vi "test_Create Periodic & Trigger Message.vi"(8 "error in (no error)":errorcluster, 11 "TestCase in":refnum<class "Instrument Addon Scripting API Messages Unit Tests.lvclass">) -> (0 "error out":errorcluster, 3 "TestCase out":refnum<class "Instrument Addon Scripting API Messages Unit Tests.lvclass">)   [LabVIEW 2019, in "Instrument Addon Scripting API Messages Unit Tests.lvclass"]
uses:
  Instrument Addon Scripting API Messages Unit Tests.lvclass
  <vilib>/addons/_JKI Toolkits/VI Tester/TestCase.llb/TestCase.lvclass
  APIs/Scripting API/Instrument Addon Scripting API.lvlib
  NationalInstruments.VeriStand.SystemDefinitionAPI
  <vilib>/NI VeriStand/Custom Device Tools/Custom Device Utility Library/Custom Device Utility Library.lvlib
  Addon/Addon Shared/SubVIs/Constants.vi
  Addon/Addon Shared/Instrument Addon Shared.lvlib
  APIs/Scripting API/TypeDefs/Protection Types.ctl
  APIs/Scripting API/TypeDefs/Message Settings.ctl
  Addon/Addon Shared/Types/FG Control.ctl
  Addon/Addon Shared/Types/Message Generation Type.ctl
  APIs/Scripting API/Messages/Create Message - Periodic & Trigger.vi
  <vilib>/NI VeriStand/Custom Device Tools/Custom Device Utility Library/NI VeriStand - Search for Item by GUID.vi
  C:/Program Files (x86)/National Instruments/LabVIEW 2019/vi.lib/addons/_JKI Toolkits/VI Tester/TestCase.llb/TestCase.lvclass
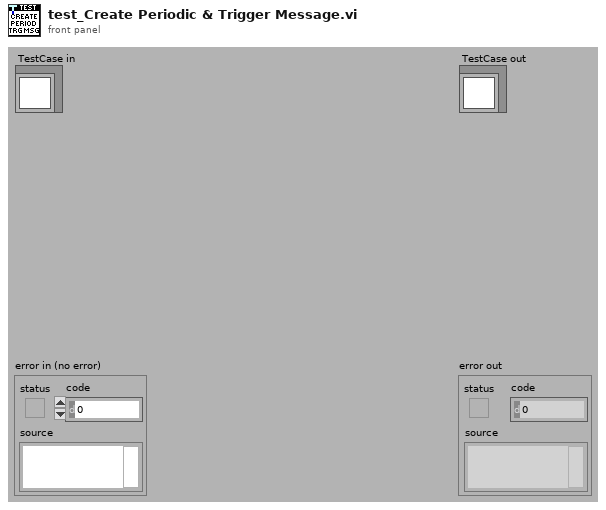
[diagram p1: front panel]
types:
  T1 = typedef "Instrument Addon Shared.lvlib/FG Control.ctl" = enum16{"Get", "Set"}
  T2 = typedef "Instrument Addon Shared.lvlib/Message Generation Type.ctl" = enum16{"Trigger Only", "Periodic & Trigger", "Value Change & Trigger"}
  T3 = typedef "Instrument Addon Scripting API.lvlib/Message Settings.ctl" = cluster{"Protection":T4, "Enable Periodic Default":bool, "Trigger Channel refnum":u64}
  T4 = typedef "Instrument Addon Scripting API.lvlib/Protection Types.ctl" = enum16{"None", "CRC-32", "Checksum U16", "Checksum U32", "Checksum U8"}
  T5 = typedef "Custom Device API.lvlib/Custom Device Item Ref.ctl" = u64
  T6 = typedef "Instrument Addon Shared.lvlib/Trigger Parameters.ctl" = cluster{"Use Channel":bool, "Channel Path":string}
  T7 = typedef "Instrument Addon Shared.lvlib/Message Parameters.ctl" = cluster{"Generation Type":T2, "Period":dbl, "Include Protection":bool, "Type":string}
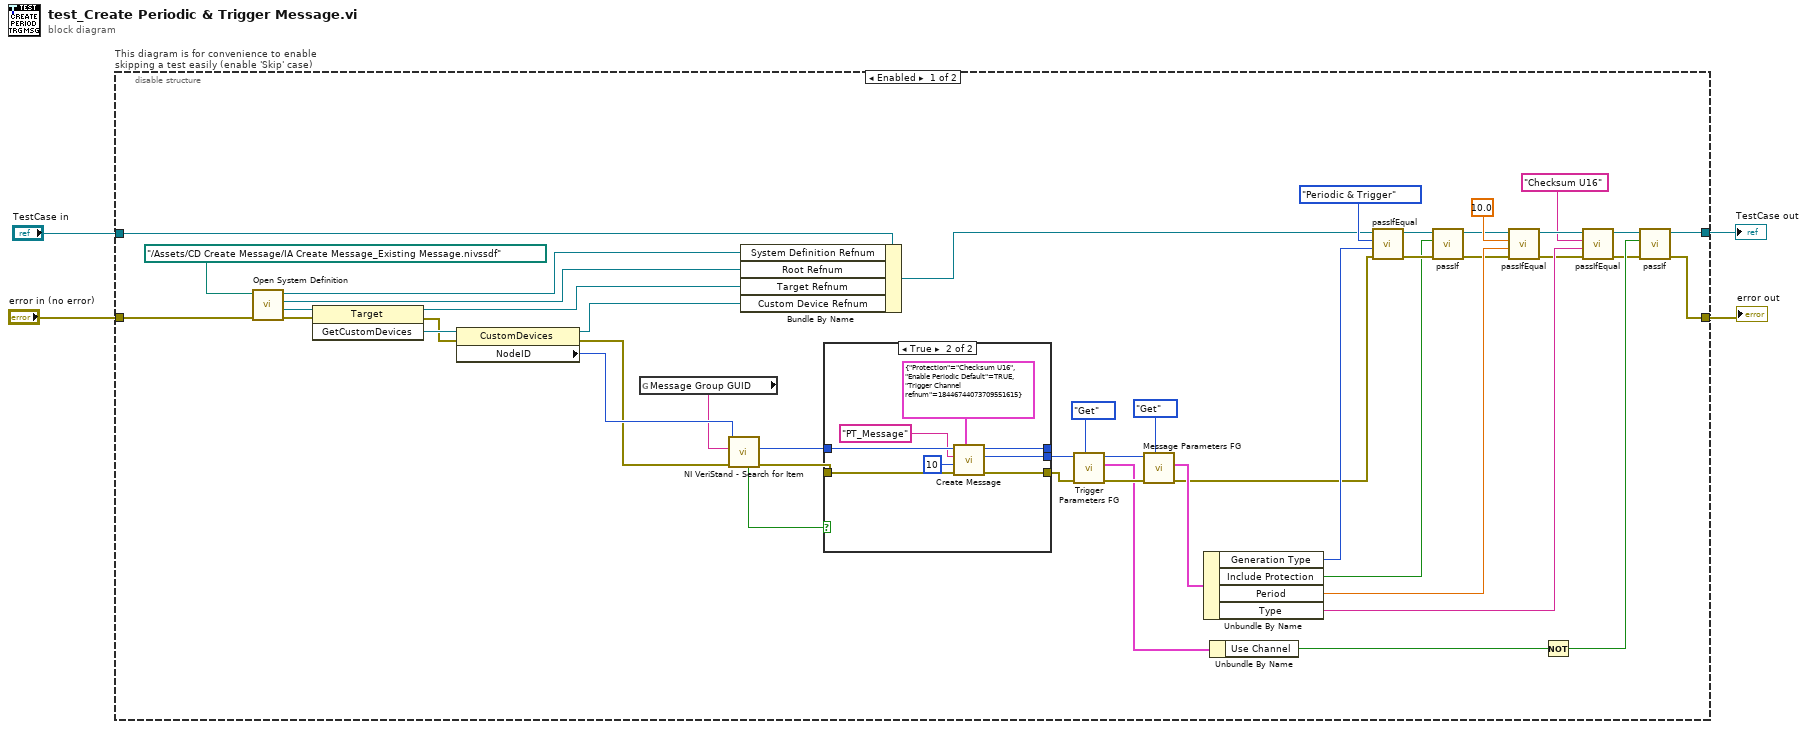
[diagram p0: block diagram]
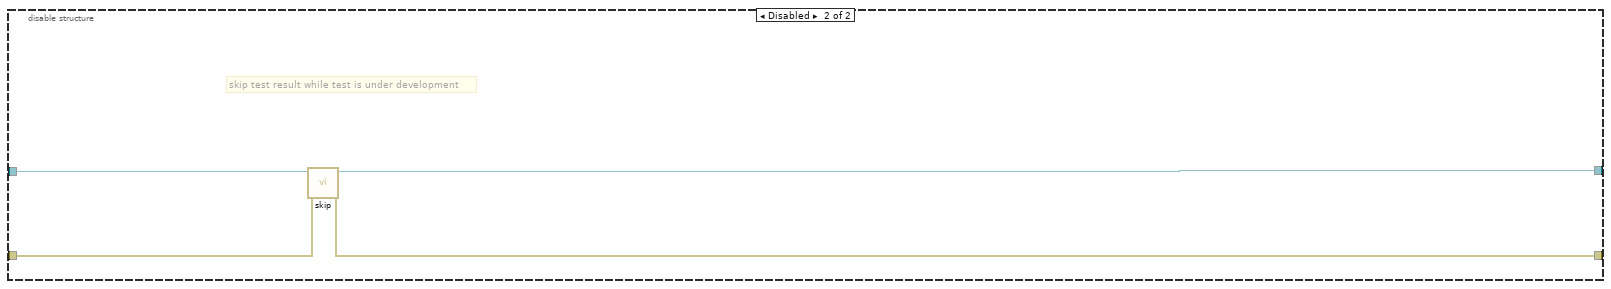
[diagram p3: hidden frame]
diagram:
  n1 = disable-structure "This diagram is for convenience to enable skipping a test easily (enable 'Skip' case)" shown="Enabled" {
    disable-tunnel: "TestCase in" -> [w10 w63]
    disable-tunnel: [w16 w61] -> w1
    disable-tunnel: [w17 w62] -> w3
    disable-tunnel: "error in (no error)" -> [w49 w60]
    frame Enabled {
      n2 = call "Open System Definition.vi"("error in (no error)"=w49, "System Definition File"=path "../Assets/CD Create Message/IA Create Message_Existing Message.nivssdf" ("SDF file")) -> ("error out"=w42:errorcluster, "Target Refnum"=w48:refnum<k24>, "Root Refnum"=w8:refnum<k24>, "System Definition Refnum"=w9:refnum<k24>)  [unwired: 6 in]
      n3 = invoke class="Target" method="GetCustomDevices"(reference=w48, error in=w42) -> (reference out=w7:refnum<k24>, error out=w41:errorcluster, "GetCustomDevices"=w47:refnum<k24>)  [unwired: 1 in]
      n4 = property class="CustomDevices"(reference=w47, error in=w41) -> (reference out=w6:refnum<k24>, error out=w40:errorcluster, "NodeID"=w46:u64)
      n5 = global read "Constants.vi" "Message Group GUID"() -> (w45:string)
      n6 = call-poly <vilib>:"NI VeriStand - Search for Item.vi"("error in"=w40, "Item GUID"=w45, "Section Ref in"=w46) -> ("error out"=w39:errorcluster, "Item Ref"=w44:T5, "Found"=w43:bool)  [unwired: 5 in, 1 out]
      n7 = Bundle By Name(cluster=w10, "System Definition Refnum"=w9, "Root Refnum"=w8, "Target Refnum"=w7, "Custom Device Refnum"=w6) -> (w5:refnum<class "Instrument Addon Scripting API Messages Unit Tests.lvclass">)
      n8 = case shown="True" w43 {
        tunnel: w44 -> [_ w59]
        tunnel: [w51 w58] -> w26
        tunnel: w39 -> [w51 w57]
        tunnel: [_ w56] -> w24
        tunnel: [_ w55] -> _
        frame False {
        }
        frame True {
          n9 = call-poly "Create Message.vi"("optional settings"=T3 {"Protection"=enum."Checksum U16", "Enable Periodic Default"=TRUE, "Trigger Channel refnum"=18446744073709551615} ("Message Settings"), "error in (no error)"=w57, "period (s)"=u32 10 ("Period"), "message name"="PT_Message", "message group refnum in"=w59) -> ("error out"=w58:errorcluster, "message refnum out"=w56:T5, "message group refnum out"=w55:T5)  [unwired: 4 in]
        }
      }
      n10 = call "Trigger Parameters FG.vi"("Action"=FG_Control."Get", "error in (no error)"=w26, "Item Ref in"=w24) -> ("error out"=w25:errorcluster, "Trigger Parameters"=w22:T6, "Item Ref out"=w23:T5)  [unwired: 6 in]
      n11 = call "Message Parameters FG.vi"("Action"=FG_Control."Get", "error in (no error)"=w25, "Item Ref in"=w23) -> ("error out"=w34:errorcluster, "Message Settings out"=w37:T7)  [unwired: 6 in, 1 out]
      n12 = Unbundle By Name(w37) -> ("Generation Type"=w36:T2, "Include Protection"=w11:bool, "Period"=w33:dbl, "Type"=w30:string)
      n13 = Unbundle By Name(w22) -> ("Use Channel"=w21:bool)
      n14 = call-dynamic "passIfEqual.vi"("error in (no error)"=w34, "y"=w36, "x"=Message_Generation_Type."Periodic & Trigger" ("Generation Type"), "TestCase in"=w5) -> ("error out"=w15:errorcluster, "TestCase out"=w13:refnum<class "Instrument Addon Scripting API Messages Unit Tests.lvclass">)  [unwired: 6 in]
      n15 = call-dynamic "passIf.vi"("error in (no error)"=w15, "pass"=w11, "TestCase in"=w13) -> ("error out"=w14:errorcluster, "TestCase out"=w12:refnum<class "Instrument Addon Scripting API Messages Unit Tests.lvclass">)  [unwired: 7 in]
      n16 = call-dynamic "passIfEqual.vi"("error in (no error)"=w14, "y"=w33, "x"=10.0 ("Period"), "TestCase in"=w12) -> ("error out"=w28:errorcluster, "TestCase out"=w31:refnum<class "Instrument Addon Scripting API Messages Unit Tests.lvclass">)  [unwired: 6 in]
      n17 = Not(x=w21) -> (.not. x?=w20:bool)
      n18 = call-dynamic "passIfEqual.vi"("error in (no error)"=w28, "y"=w30, "x"="Checksum U16" ("Type"), "TestCase in"=w31) -> ("error out"=w19:errorcluster, "TestCase out"=w18:refnum<class "Instrument Addon Scripting API Messages Unit Tests.lvclass">)  [unwired: 6 in]
      n19 = call-dynamic "passIf.vi"("error in (no error)"=w19, "pass"=w20, "TestCase in"=w18) -> ("error out"=w17:errorcluster, "TestCase out"=w16:refnum<class "Instrument Addon Scripting API Messages Unit Tests.lvclass">)  [unwired: 7 in]
    }
    frame Disabled {
      # "skip test result while test is under development"
      n20 = call <vilib>:"skip.vi"("error in (no error)"=w60, "TestCase in"=w63) -> ("error out"=w62:errorcluster, "TestCase out"=w61:refnum<class "Instrument Addon Scripting API Messages Unit Tests.lvclass">)  [unwired: 8 in]
    }
  }
  "error out" <- w3
  "TestCase out" <- w1
